vi "boundry.vi"() -> ()   [LabVIEW 2013]
uses:
  <vilib>/NXT/Block Support/NXT_OutputPort.ctl
  <vilib>/NXT/Block Support/NXT_InputPort.ctl
  <vilib>/NXT/NXTIO Xnodes/NXTIONodeSubVIs/NXTStopMotors.vi
  <vilib>/NXT/Dual Mode Library/Sensors/EV3_Gyro_Angle.vi
  <vilib>/NXT/Subs/LVHSConnector.ctl
  <vilib>/NXT/NXTIO Xnodes/AddressXNode/NXTIOAddress.xnode
  <vilib>/NXT/NXTIO Xnodes/NXTIOXNode/NXTIO.xnode
  <vilib>/NXT/LegoClasses/BrickReference/BrickReference.lvclass
panel:
  out "Degrees":sgl
  out "rightB":dbl
  out "leftA":dbl
  out "left":bool
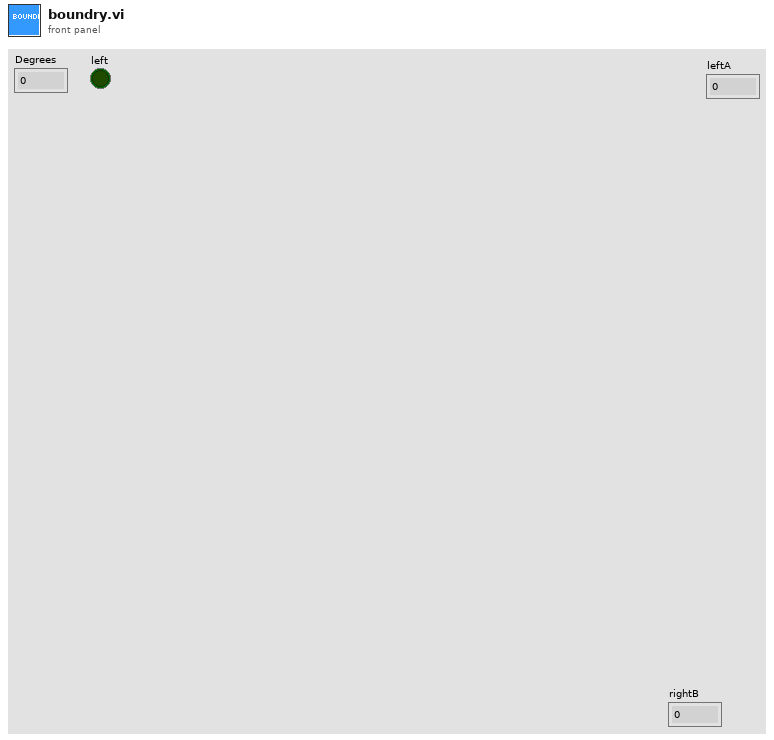
[diagram p1: front panel]
types:
  T1 = typedef "NXT_OutputPort.ctl" = u8
  T2 = typedef "NXT_InputPort.ctl" = u32
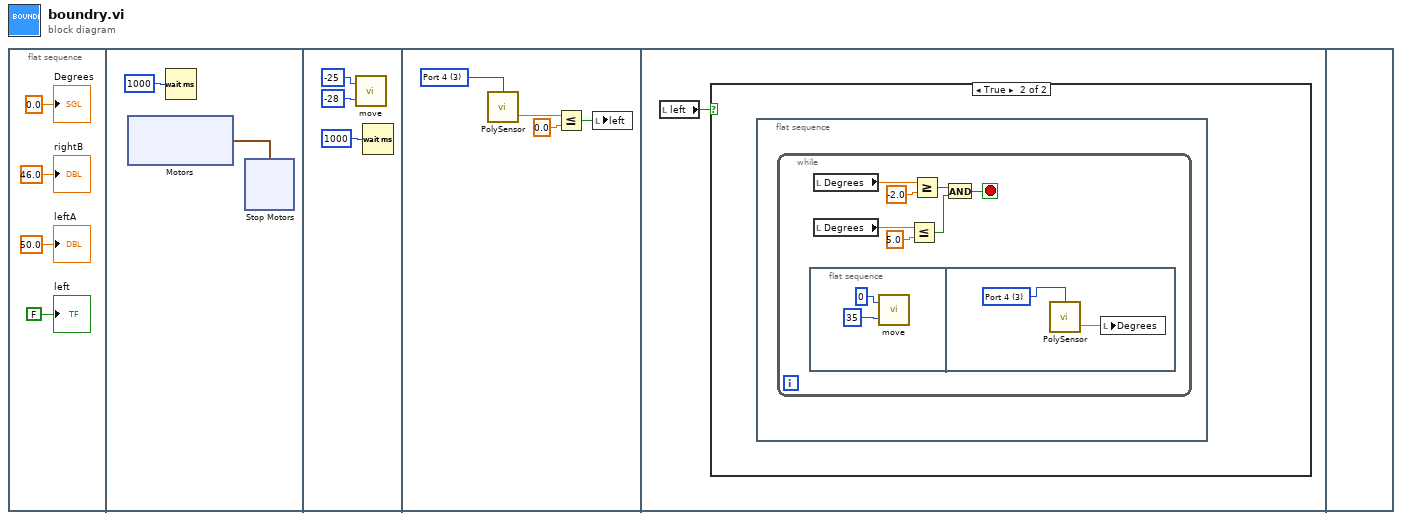
[diagram p0: block diagram]
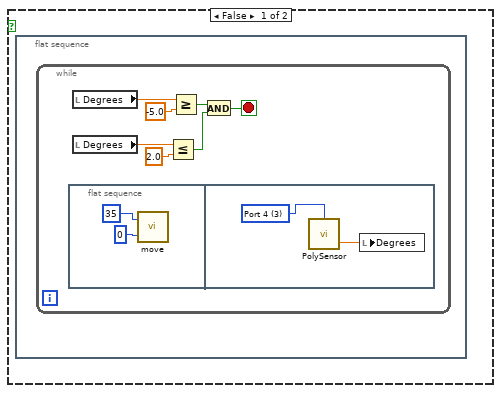
[diagram p2: hidden frame]
diagram:
  n1 = flat-sequence {
    frame #0 {
      "leftA" <- 50.0 ("leftA")
      "rightB" <- 46.0 ("Numeric")
      "Degrees" <- sgl 0.0 ("Degrees")
      "left" <- FALSE ("left")
    }
    frame #1 {
      n2 = xnode "Motors"() -> ("Motor"=w6:cluster{"Port":T1, "Port":T1})
      n3 = Wait (ms)(milliseconds to wait=u32 1000) -> ()  [unwired: 1 out]
      n4 = xnode "Stop Motors"("Motors"=w6) -> ()  [unwired: 1 in, 1 out]
    }
    frame #2 {
      n5 = call "move.vi"("speedLeft"=i8 -28, "speedRight"=i8 -25) -> ()  [unwired: 1 in]
      n6 = Wait (ms)(milliseconds to wait=u32 1000) -> ()  [unwired: 1 out]
    }
    frame #3 {
      w19 = T2 3 items=["Port 1", "Port 2", "Port 3", "Port 4"] ("Port (Port 1)")
      n7 = call-poly <vilib>:"PolySensor.vi"("Port (Port 1)"=w19) -> ("Degrees"=w18:sgl)  [unwired: 2 in, 1 out]
      n8 = Less Or Equal?(x=w18, y=sgl 0.0) -> (x <= y?=w16:bool)
      n9 = local write "left"(w16) -> ()
    }
    frame #4 {
      n10 = local read "left"() -> (w20:bool)
      n11 = case shown="True" w20 {
        frame False {
          n12 = flat-sequence {
            frame #0 {
              n13 = while {
                stop <- w27 stop-if-true
                n14 = flat-sequence {
                  frame #0 {
                    n15 = call "move.vi"("speedLeft"=i8 0, "speedRight"=i8 35) -> ()  [unwired: 1 in]
                  }
                  frame #1 {
                    w30 = T2 3 items=["Port 1", "Port 2", "Port 3", "Port 4"] ("Port (Port 1)")
                    n16 = call-poly <vilib>:"PolySensor.vi"("Port (Port 1)"=w30) -> ("Degrees"=w31:sgl)  [unwired: 2 in, 1 out]
                    n17 = local write "Degrees"(w31) -> ()
                  }
                }
                n18 = local read "Degrees"() -> (w22:sgl)
                n19 = local read "Degrees"() -> (w21:sgl)
                n20 = Less Or Equal?(x=w21, y=2.0) -> (x <= y?=w25:bool)
                n21 = Greater Or Equal?(x=w22, y=-5.0) -> (x >= y?=w26:bool)
                n22 = And(x=w26, y=w25) -> (x .and. y?=w27:bool)
              }
            }
          }
        }
        frame True {
          n23 = flat-sequence {
            frame #0 {
              n24 = while {
                stop <- w38 stop-if-true
                n25 = flat-sequence {
                  frame #0 {
                    n26 = call "move.vi"("speedLeft"=i8 35, "speedRight"=i8 0) -> ()  [unwired: 1 in]
                  }
                  frame #1 {
                    w41 = T2 3 items=["Port 1", "Port 2", "Port 3", "Port 4"] ("Port (Port 1)")
                    n27 = call-poly <vilib>:"PolySensor.vi"("Port (Port 1)"=w41) -> ("Degrees"=w42:sgl)  [unwired: 2 in, 1 out]
                    n28 = local write "Degrees"(w42) -> ()
                  }
                }
                n29 = local read "Degrees"() -> (w33:sgl)
                n30 = local read "Degrees"() -> (w32:sgl)
                n31 = Less Or Equal?(x=w32, y=5.0) -> (x <= y?=w36:bool)
                n32 = Greater Or Equal?(x=w33, y=-2.0) -> (x >= y?=w37:bool)
                n33 = And(x=w37, y=w36) -> (x .and. y?=w38:bool)
              }
            }
          }
        }
      }
    }
    frame #5 {
    }
  }
